vi "Xml_Write_Disk.vi"(8 "error in (no error)":errorcluster, 10 "XML Name":string, 11 "Spectrum Path":path) -> (0 "error out":errorcluster, 3 "Path out":path)   [LabVIEW 2024]
uses:
  Global_Variables.vi
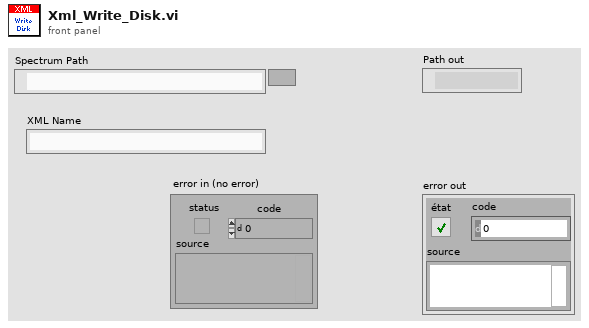
[diagram p1: front panel]
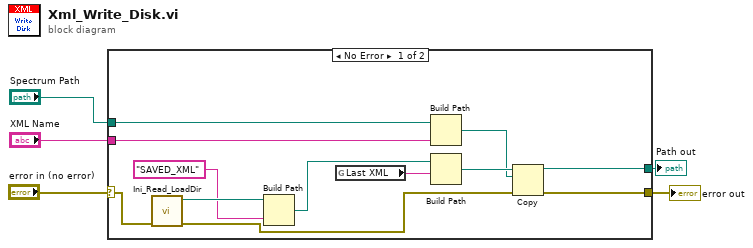
[diagram p0: block diagram]
diagram:
  n1 = case shown="No Error" "error in (no error)" {
    selector: "error in (no error)" -> [w12 w19]
    tunnel: [w7 w18] -> w1
    tunnel: [w6 w19] -> w2
    tunnel: "XML Name" -> [w15 _]
    tunnel: "Spectrum Path" -> [w14 w18]
    frame No Error {
      n2 = call "Ini_Read_LoadDir.vi"("error in (no error)"=w12) -> ("error out"=w9:errorcluster, "Path"=w10:path)  [unwired: 9 in]
      n3 = Build Path(base path=w10, name or relative path="SAVED_XML") -> (appended path=w11:path)
      n4 = global read "Global_Variables.vi" "Last XML"() -> (w13:string)
      n5 = Build Path(base path=w14, name or relative path=w15) -> (appended path=w16:path)
      n6 = Build Path(base path=w11, name or relative path=w13) -> (appended path=w17:path)
      n7 = Copy(8:w9, 10:w16, 11:w17) -> (0:w6:errorcluster, 3:w7:path)  [unwired: 2 in, 1 out]
    }
    frame Error {
    }
  }
  "error out" <- w2
  "Path out" <- w1
